vi "sos.vi"(7 "bypass":bool, 8 "input valid":bool=TRUE, 9 "b":fxp<+/-,24,8>[](array[numeric])=[0.0, 0.0, 0.0], 10 "anot":fxp<+/-,24,8>[](array[numeric])=[0.0, 0.0], 11 "input":fxp<+/-,26,9>) -> (0 "ready for input":bool, 1 "output valid":bool, 3 "output":fxp<+/-,26,9>)   [LabVIEW 2016]
uses:
  <vilib>/rvi/FXPMathLib/FxpMul/XNode/nifxpmath_Multiplier.xnode
  <vilib>/rvi/FXPMathLib/FxpAdd/XNode/nifxpmath_Add.xnode
  <vilib>/rvi/FXPMathLib/sim/FxpSim.dll
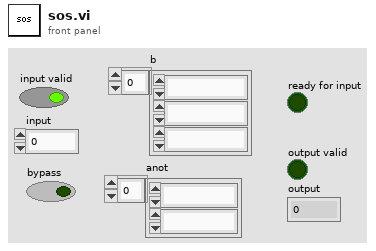
[diagram p1: front panel]
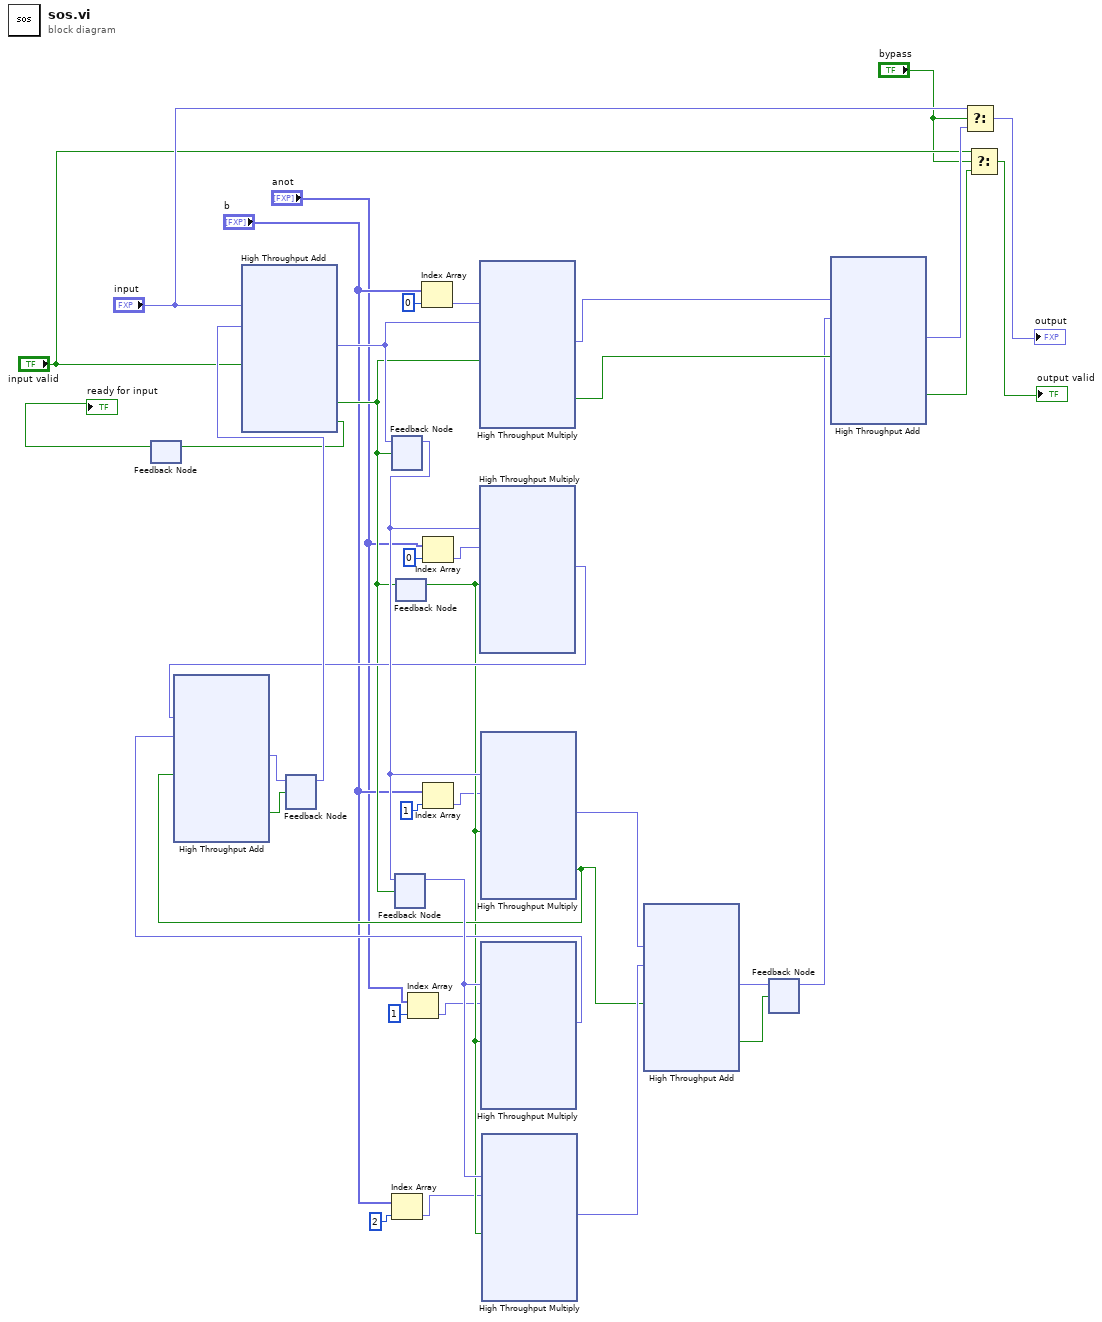
[diagram p0: block diagram]
diagram:
  n1 = feedback #1() -> (→"ready for input":bool)  [unwired: 1 in]
  n2 = feedback #2() -> (w33:fxp<+/-,36,16>)  [unwired: 1 in]
  n3 = xnode ("High Throughput Add")("x"="input", "y"=w33, "input valid"="input valid") -> ("x+y"=w37:fxp<+/-,36,16>, "output valid"=w27:bool, "ready for input"=w25:bool)  [unwired: 1 in]
  n4 = feedback-in #1(w25) -> ()
  n5 = feedback #3() -> (w39:fxp<+/-,36,16>)  [unwired: 1 in]
  n6 = feedback-in #3(w37, w27) -> ()
  n7 = Index Array(array="b", index=2) -> (element=w13:fxp<+/-,24,8>)
  n8 = feedback #4() -> (w38:fxp<+/-,36,16>)  [unwired: 1 in]
  n9 = feedback-in #4(w39, w27) -> ()
  n10 = feedback #5() -> (w26:bool)  [unwired: 1 in]
  n11 = feedback-in #5(w27) -> ()
  n12 = Index Array(array="anot", index=1) -> (element=w9:fxp<+/-,24,8>)
  n13 = Index Array(array="b", index=0) -> (element=w18:fxp<+/-,24,8>)
  n14 = Index Array(array="anot", index=0) -> (element=w11:fxp<+/-,24,8>)
  n15 = Index Array(array="b", index=1) -> (element=w17:fxp<+/-,24,8>)
  n16 = xnode ("High Throughput Multiply")("x"=w18, "y"=w37, "input valid"=w27) -> ("x*y"=w23:fxp<+/-,36,16>, "output valid"=w22:bool)  [unwired: 1 in, 1 out]
  n17 = xnode ("High Throughput Multiply")("x"=w39, "y"=w11, "input valid"=w26) -> ("x*y"=w32:fxp<+/-,36,16>)  [unwired: 1 in, 2 out]
  n18 = xnode ("High Throughput Multiply")("x"=w39, "y"=w17, "input valid"=w26) -> ("x*y"=w31:fxp<+/-,36,16>, "output valid"=w29:bool)  [unwired: 1 in, 1 out]
  n19 = xnode ("High Throughput Multiply")("x"=w38, "y"=w9, "input valid"=w26) -> ("x*y"=w36:fxp<+/-,36,16>)  [unwired: 1 in, 2 out]
  n20 = xnode ("High Throughput Add")("x"=w32, "y"=w36, "input valid"=w29) -> ("x+y"=w35:fxp<+/-,36,16>, "output valid"=w34:bool)  [unwired: 1 in, 1 out]
  n21 = feedback-in #2(w35, w34) -> ()
  n22 = xnode ("High Throughput Multiply")("x"=w38, "y"=w13, "input valid"=w26) -> ("x*y"=w30:fxp<+/-,36,16>)  [unwired: 1 in, 2 out]
  n23 = xnode ("High Throughput Add")("x"=w31, "y"=w30, "input valid"=w29) -> ("x+y"=w28:fxp<+/-,36,16>, "output valid"=w20:bool)  [unwired: 1 in, 1 out]
  n24 = feedback #6() -> (w21:fxp<+/-,36,16>)  [unwired: 1 in]
  n25 = feedback-in #6(w28, w20) -> ()
  n26 = xnode ("High Throughput Add")("x"=w23, "y"=w21, "input valid"=w22) -> ("x+y"=w6:fxp<+/-,26,9>, "output valid"=w3:bool)  [unwired: 1 in, 1 out]
  n27 = Select(t="input", s="bypass", f=w6) -> (s? t:f=→"output":fxp<+/-,26,9>)
  n28 = Select(t="input valid", s="bypass", f=w3) -> (s? t:f=→"output valid":bool)
